vi "Write Curent source results.vi"(8 "error in (no error)":errorcluster, 10 "Curent source results":refnum<class "Acquired Result.lvclass">[](array[class]), 11 "IV in":refnum<class "IV.lvclass">) -> (0 "error out":errorcluster, 3 "IV out":refnum<class "IV.lvclass">)   [LabVIEW 2021, in "IV.lvclass"]
uses:
  IV.lvclass
  Libraries/Instruments/Results/Acquired Result/Acquired Result.lvclass
  IV.lvclass/IV.ctl
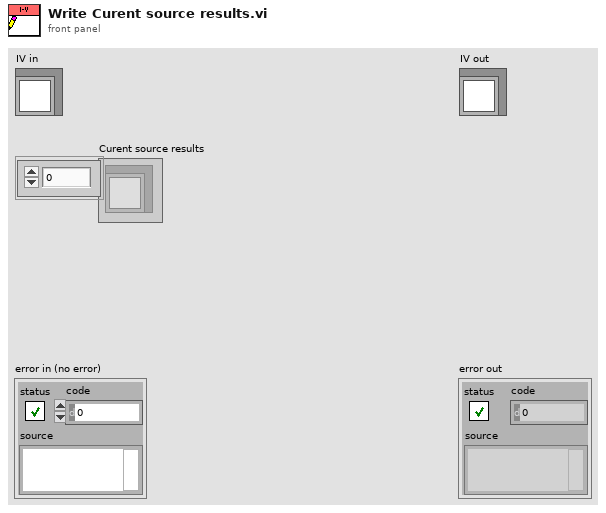
[diagram p1: front panel]
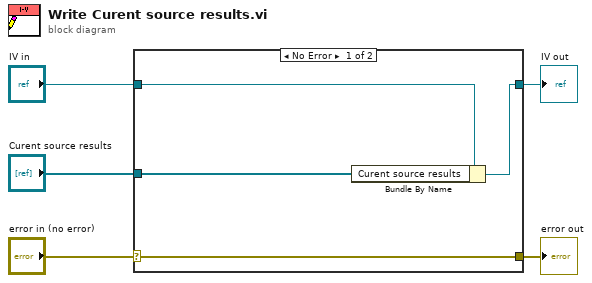
[diagram p0: block diagram]
diagram:
  n1 = case shown="No Error" "error in (no error)" {
    selector: "error in (no error)" -> [w9 w10]
    tunnel: [w9 w10] -> w4
    tunnel: [w7 w11] -> w2
    tunnel: "IV in" -> [w8 w11]
    tunnel: "Curent source results" -> [w6 _]
    frame No Error {
      n2 = Bundle By Name(cluster=w8, "Curent source results"=w6) -> (w7:refnum<class "IV.lvclass">)
    }
    frame Error {
    }
  }
  "error out" <- w4
  "IV out" <- w2
